vi "Facade.vi"(0 "Data In":T6, 2 "Display State In":T2={"Hierarchy"=[], "File/Directory Path"=path "", "Relative File Paths"=[], "Hide Undefined Channels"=FALSE, "Static File Structure"=FALSE, "Filtering"={"Filtered Groups"=[], "Group Filter Mode"=enum."Exclude", "Group Filter Regex?"=FALSE, "Filtered Channels"=[], "Channel Filter Mode"=enum."Exclude", "Channel Filter Regex?"=FALSE, "Filter Time Start"=timestamp(0 s since 1904-01-01), "Filter Time End"=timestamp(0 s since 1904-01-01), "Time Filter Mode"=enum."Include", "Time Filter Enabled"=FALSE}, "File Contents Tree"=refnum, "Properties Table"=refnum, "Loading Indicator"=refnum}, 3 "Container State":T5) -> (6 "Data Out":T6, 7 "Display State Out":T2={"Hierarchy"=[], "File/Directory Path"=path "", "Relative File Paths"=[], "Hide Undefined Channels"=FALSE, "Static File Structure"=FALSE, "Filtering"={"Filtered Groups"=[], "Group Filter Mode"=enum."Exclude", "Group Filter Regex?"=FALSE, "Filtered Channels"=[], "Channel Filter Mode"=enum."Exclude", "Channel Filter Regex?"=FALSE, "Filter Time Start"=timestamp(0 s since 1904-01-01), "Filter Time End"=timestamp(0 s since 1904-01-01), "Time Filter Mode"=enum."Include", "Time Filter Enabled"=FALSE}, "File Contents Tree"=refnum, "Properties Table"=refnum, "Loading Indicator"=refnum}, 8 "Action":T1)   [LabVIEW 2017, in "XTree.xctl"]
uses:
  <vilib>/addons/_NIFileIO/XTree/XTree.xctl
  <vilib>/addons/_NIFileIO/XTree/Data.ctl
  <vilib>/_xctls/Container State.ctl
  <vilib>/addons/_NIFileIO/XTree/State.ctl
  <vilib>/addons/_NIFileIO/XTree/Controls/Filter Settings.ctl
  <vilib>/addons/_NIFileIO/XTree/Controls/Filter Mode.ctl
  <vilib>/_xctls/Action.ctl
  <vilib>/Utility/miscctls.llb/LVRowAndColumnTypeDef.ctl
  <vilib>/_xctls/XControlSupport.lvlib
panel:
  out "Loading Indicator":string="Loading Tree Data..."
  in  "File Contents Tree":string(tree)
  out "Properties Table":string[][](table)
  # "1. Drop the controls that make up the appearance\nof the XControl here.\n\n2. Resize the window to fit the controls\n\n3. If the XControl is of fixed size,  make the \n window not resizable from VI Properties->Window Appearance.\n\n4. If you want the controls to automatically size when the XControl sizes, check  \"Scale all objects on front panel when window resizes\" in File->VI Properties->Window Size page.\n\n5. Show the block diagram and handle events for the controls on this panel."
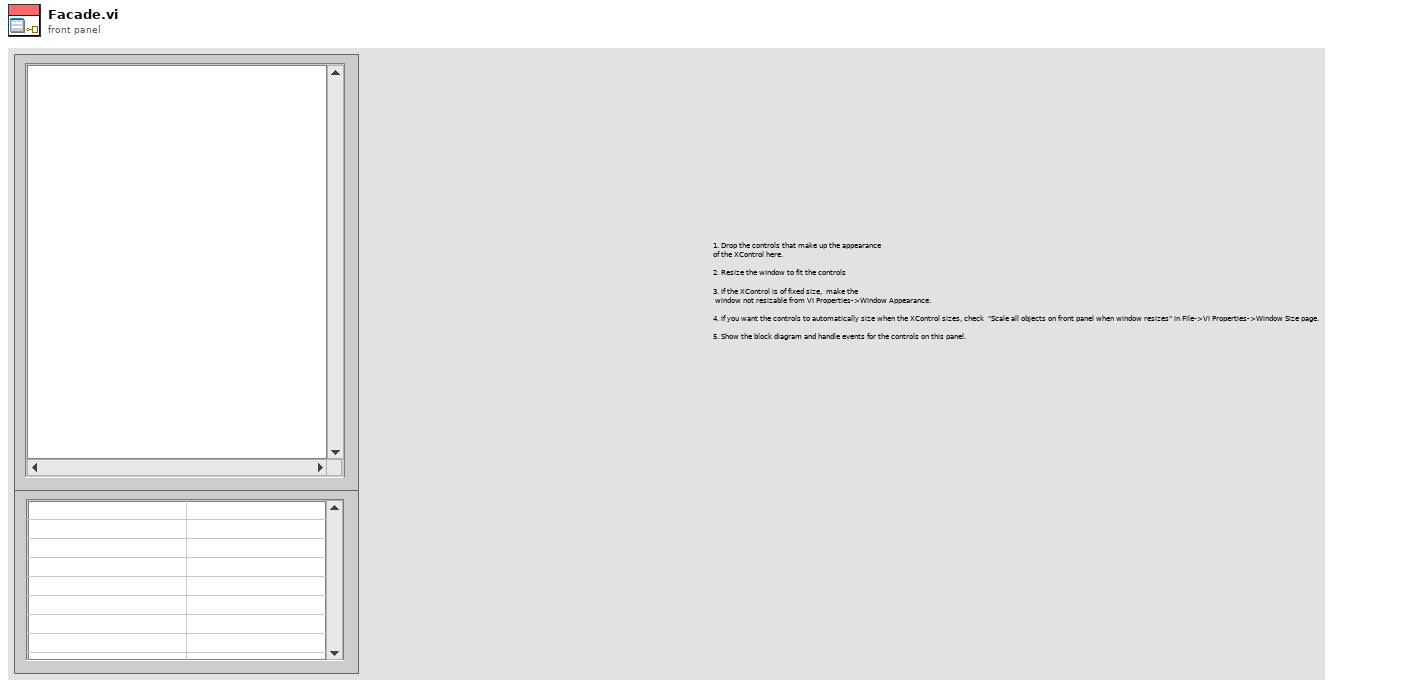
[diagram p1: front panel]
types:
  T1 = typedef "XControlSupport.lvlib/Action.ctl" = cluster{"Data Changed?":bool, "State Changed?":bool, "Action Name":string}
  T2 = typedef "XTree.xctl/State.ctl" = cluster{"Hierarchy":string[], "File/Directory Path":path, "Relative File Paths":string[], "Hide Undefined Channels":bool, "Static File Structure":bool, "Filtering":T3, "File Contents Tree":refnum<vi>, "Properties Table":refnum<vi>, "Loading Indicator":refnum<vi>}
  T3 = typedef "XTree.xctl/Filter Settings.ctl" = cluster{"Filtered Groups":string[], "Group Filter Mode":T4, "Group Filter Regex?":bool, "Filtered Channels":string[], "Channel Filter Mode":T4, "Channel Filter Regex?":bool, "Filter Time Start":timestamp, "Filter Time End":timestamp, "Time Filter Mode":T4, "Time Filter Enabled":bool}
  T4 = typedef "XTree.xctl/Filter Mode.ctl" = enum16{"Exclude", "Include"}
  T5 = typedef "XControlSupport.lvlib/Container State.ctl" = cluster{"Indicator?":bool, "Run Mode?":bool, " Refnum":refnum<vi>}
  T6 = typedef "XTree.xctl/Data.ctl" = variant
  T7 = typedef "LVRowAndColumnTypeDef.ctl" = cluster{"Row":i32, "Column":i32}
  T8 = enum16{"open", "open or create", "create or replace", "create", "open (read-only)"}
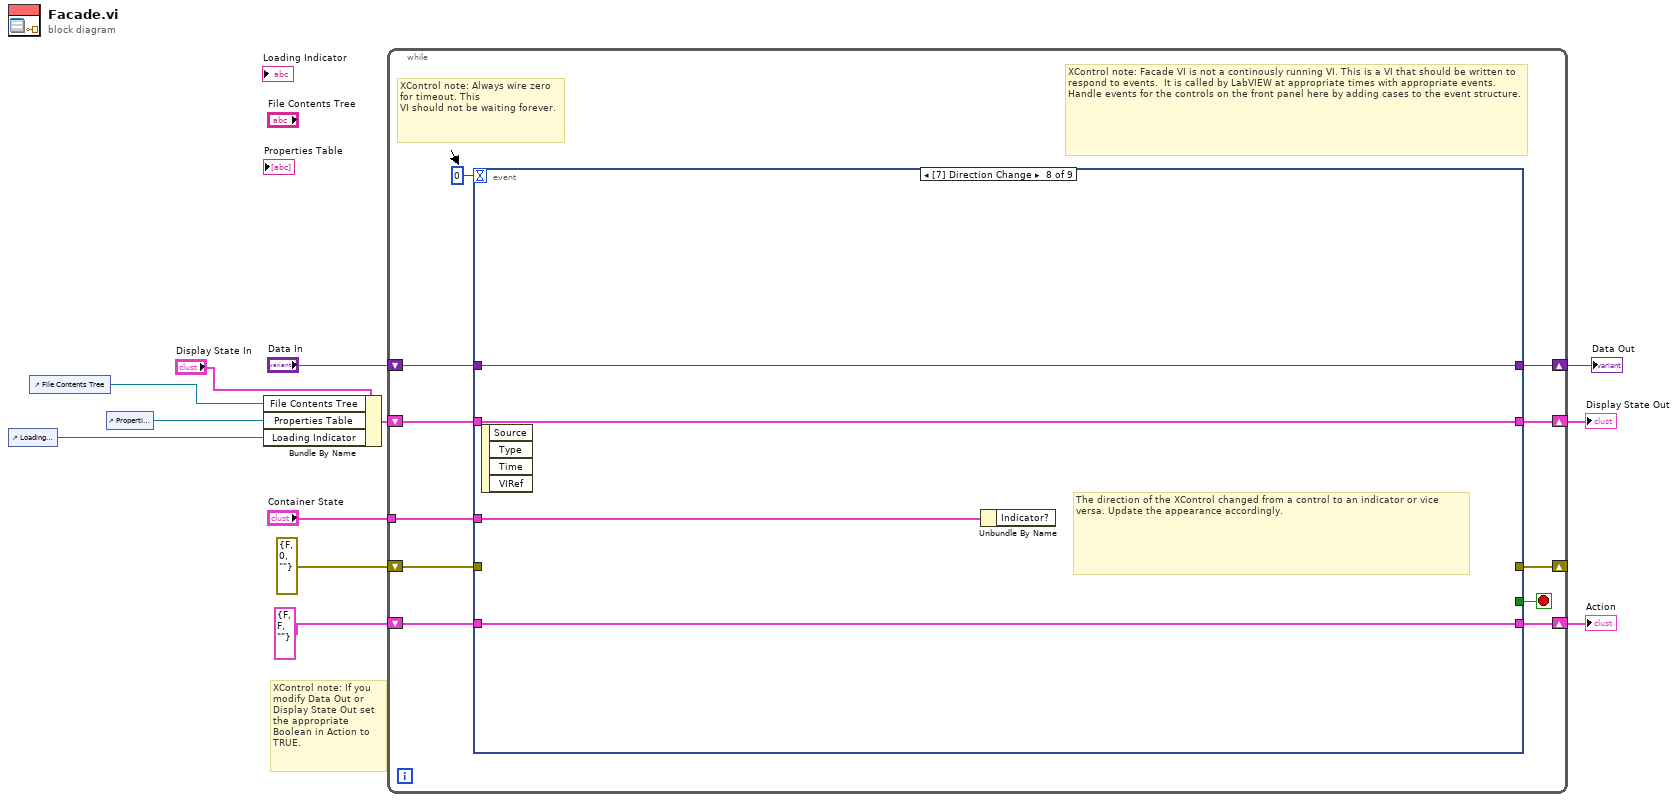
[diagram p0: block diagram]
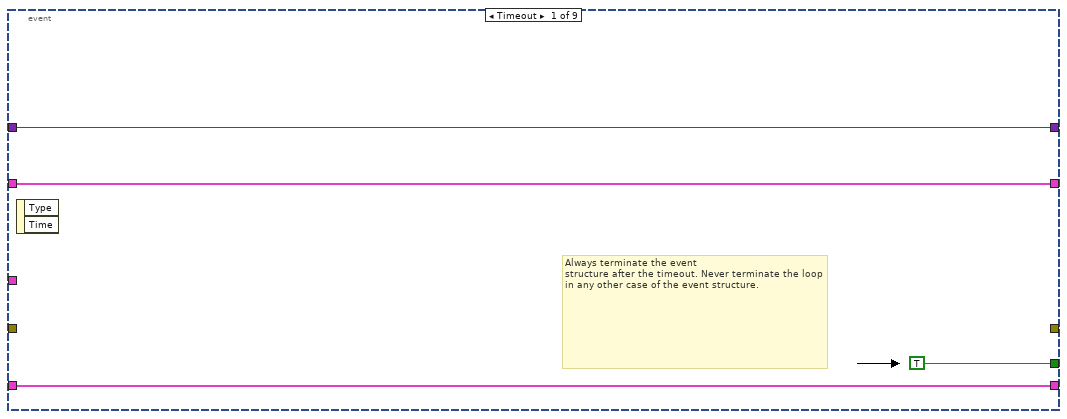
[diagram p2: hidden frame]
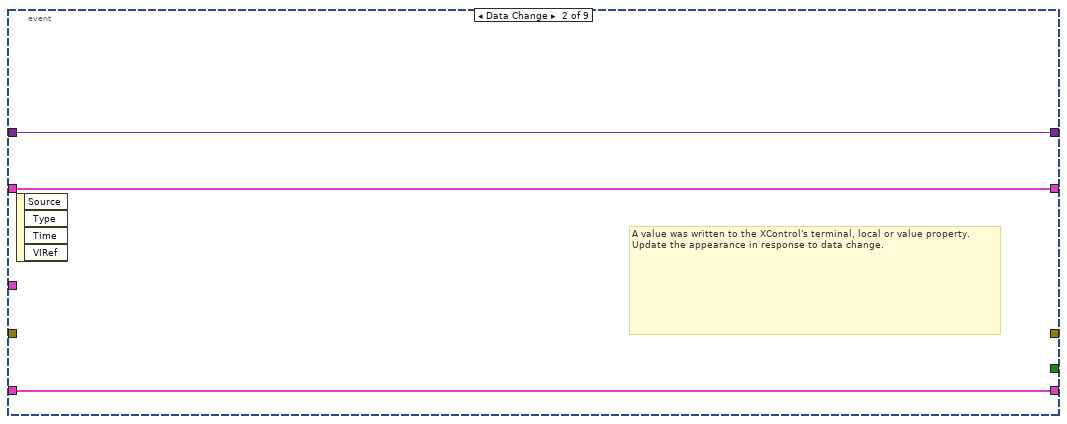
[diagram p3: hidden frame]
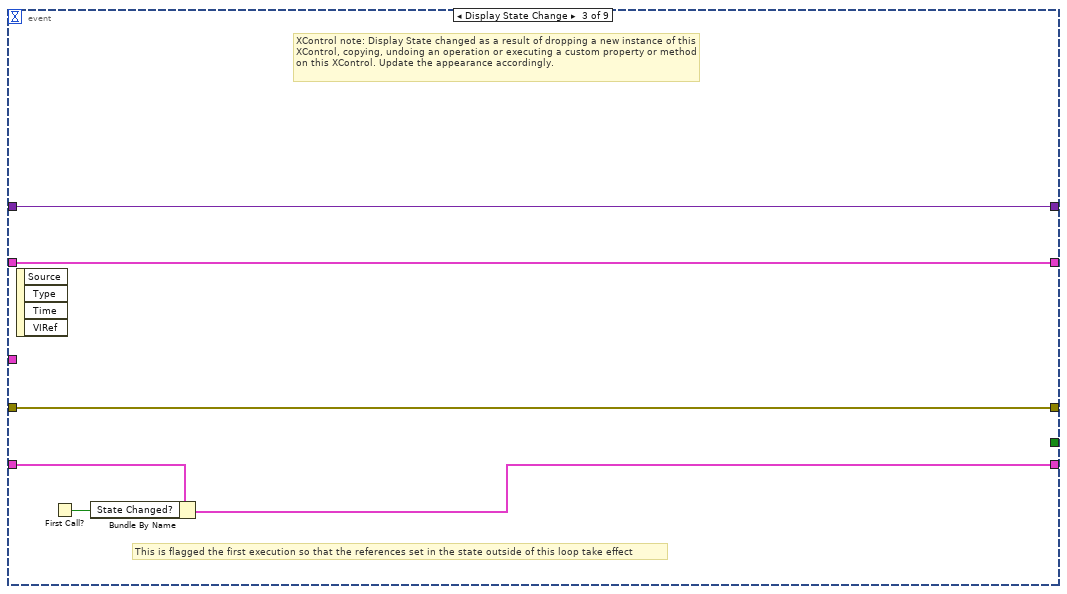
[diagram p4: hidden frame]
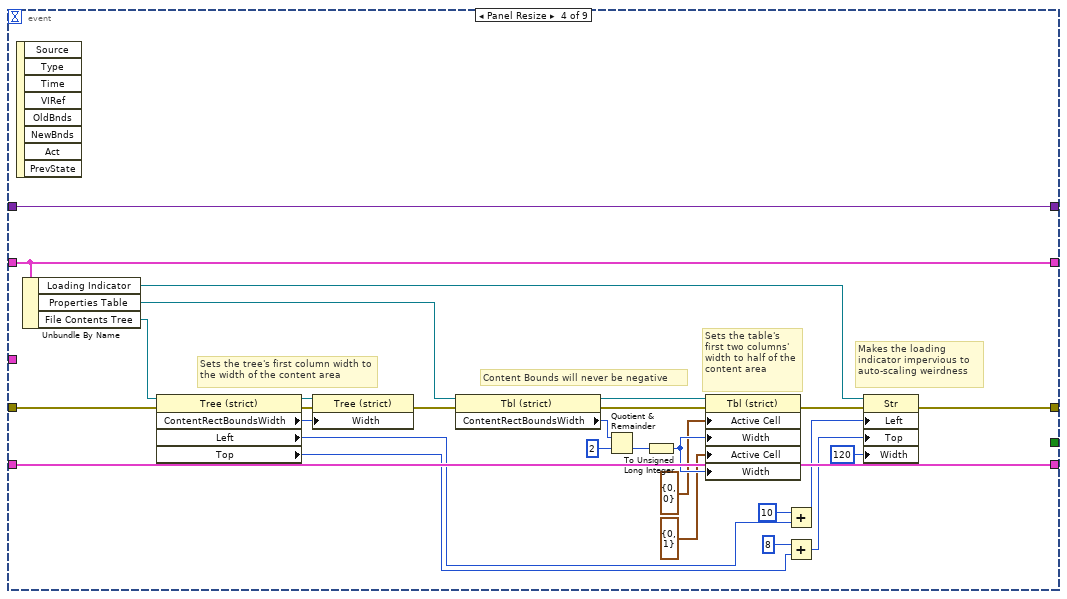
[diagram p5: hidden frame]
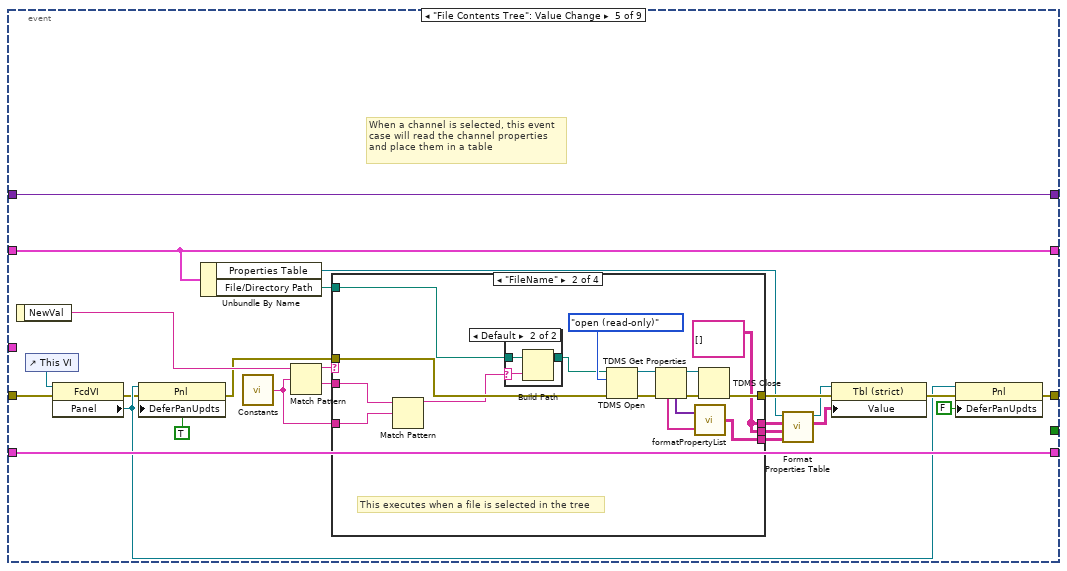
[diagram p6: hidden frame]
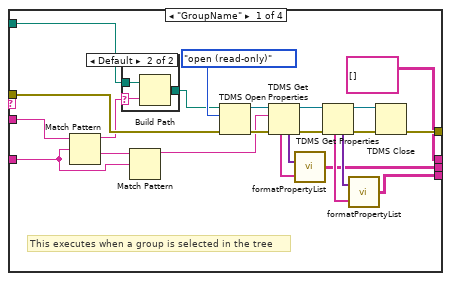
[diagram p7: hidden frame]
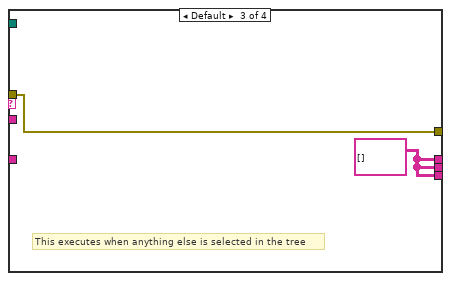
[diagram p10: hidden frame]
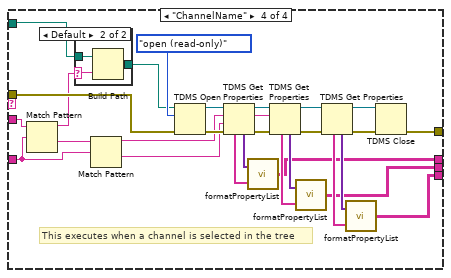
[diagram p11: hidden frame]
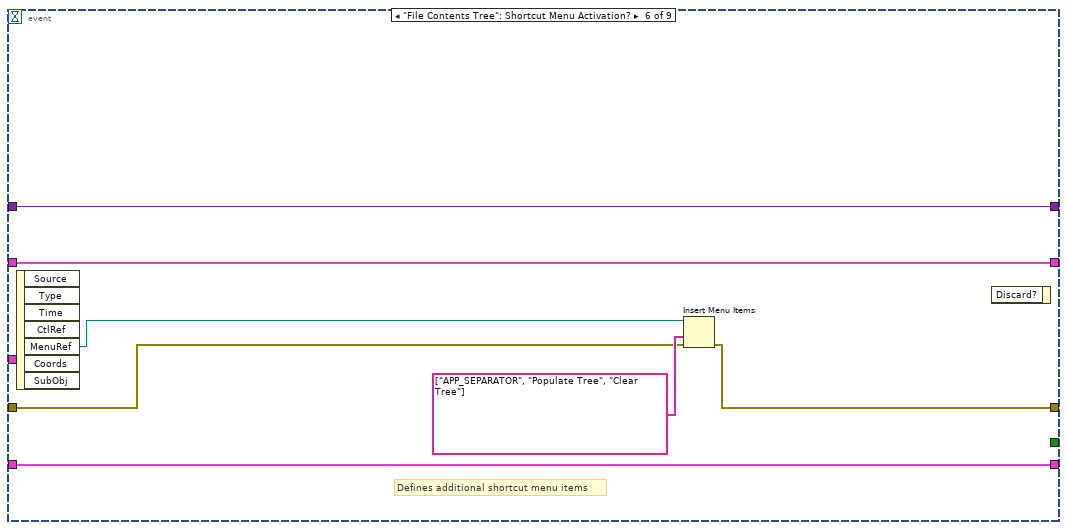
[diagram p13: hidden frame]
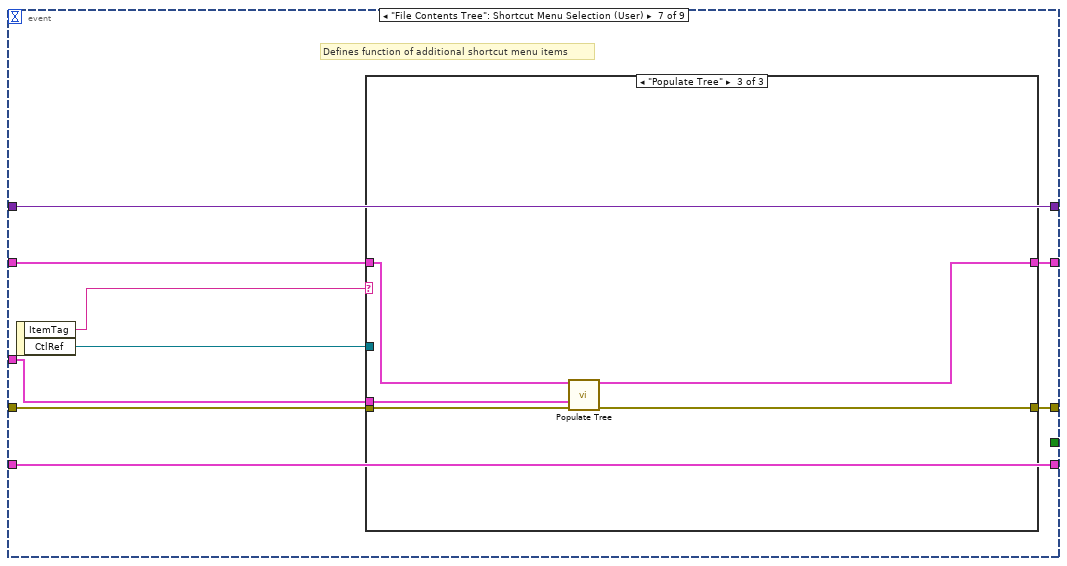
[diagram p14: hidden frame]
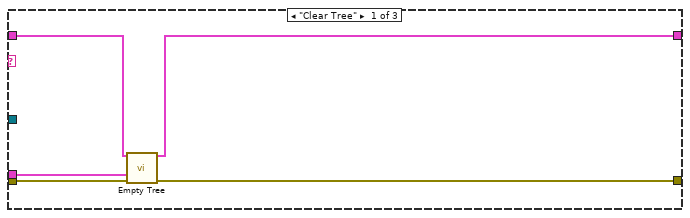
[diagram p15: hidden frame]
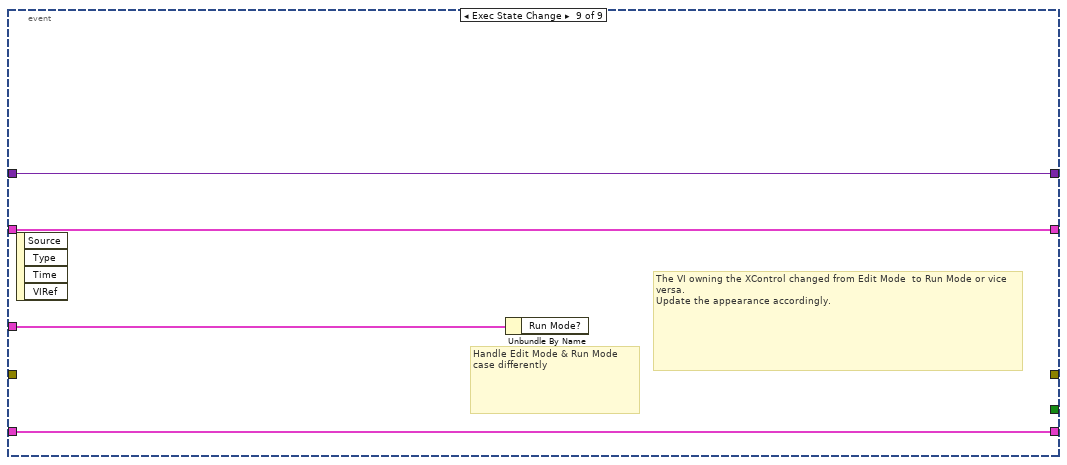
[diagram p17: hidden frame]
diagram:
  # "XControl note: If you modify Data Out or Display State Out set the appropriate Boolean in Action to TRUE."
  n1 = control-ref of="Loading Indicator"() -> (w1:refnum<vi>)
  n2 = control-ref of="File Contents Tree"() -> (w4:refnum<vi>)
  n3 = control-ref of="Properties Table"() -> (w5:refnum<vi>)
  n4 = Bundle By Name(cluster="Display State In", "File Contents Tree"=w4, "Properties Table"=w5, "Loading Indicator"=w1) -> (w2:T2)
  n5 = while {
    shift-right: [w22] -> w9
    shift-left: w2 -> [w23]
    tunnel: "Container State" -> [w19]
    shift-right: [w17] -> w12
    shift-left: "Data In" -> [w18]
    shift-right: [w15] -> w8
    shift-left: T1 {"Data Changed?"=FALSE, "State Changed?"=FALSE, "Action Name"=""} ("Action") -> [w16]
    shift-right: [w13] -> _
    shift-left: errorcluster {"status"=FALSE, "code"=0, "source"=""} ("error constant") -> [w14]
    stop <- w21 stop-if-true
    # "XControl note: Facade VI is not a continously running VI. This is a VI that should be written to respond to events.  It is called by LabVIEW at appropriate times with appropriate events. Handle events for the controls on the front panel here by adding cases to the event structure."
    # "XControl note: Always wire zero for timeout. This\nVI should not be waiting forever."
    n6 = event shown="[7] Direction Change" {
      selector: _ -> [_ _ _ _ _ _ _ _ _]
      dyn-events: _ -> [_ _ _ _ _ _ _ _ _]
      timeout: 0 -> [_ _ _ _ _ _ _ _ _]
      tunnel: w23 -> [w25 w29 w32 w52 w84 w177 w183 w201 w205]
      tunnel: [w25 w29 w32 w52 w84 w177 w180 w201 w205] -> w22
      tunnel: [TRUE _ _ _ _ _ _ _ _] -> w21
      tunnel: w19 -> [_ _ _ _ _ _ w182 w202 w206]
      tunnel: w18 -> [w24 w30 w35 w64 w88 w176 w186 w200 w204]
      tunnel: [w24 w30 w35 w64 w88 w176 w186 w200 w204] -> w17
      tunnel: [w26 w28 w33 w63 w75 w175 w185 w199 w203] -> w15
      tunnel: w16 -> [w26 w28 w36 w63 w75 w175 w185 w199 w203]
      tunnel: w14 -> [_ _ w34 w59 w66 w172 w184 _ _]
      tunnel: [_ _ w34 w45 w69 w171 w181 _ _] -> w13
      event Timeout {
        # "Always terminate the event\nstructure after the timeout. Never terminate the loop in any other case of the event structure."
        n7 = event-data() -> ()  [unwired: 1 in, 2 out]
      }
      event Data Change {
        # "A value was written to the XControl's terminal, local or value property.\nUpdate the appearance in response to data change."
        n8 = event-data() -> ()  [unwired: 1 in, 4 out]
      }
      event Display State Change {
        # "This is flagged the first execution so that the references set in the state outside of this loop take effect"
        # "XControl note: Display State changed as a result of dropping a new instance of this XControl, copying, undoing an operation or executing a custom property or method on this XControl. Update the appearance accordingly."
        n9 = event-data() -> ()  [unwired: 1 in, 4 out]
        n10 = First Call?() -> (First Call?: T/F=w31:bool)
        n11 = Bundle By Name(cluster=w36, "State Changed?"=w31) -> (w33:T1)
      }
      event Panel Resize {
        # "Makes the loading indicator impervious to auto-scaling weirdness"
        # "Sets the table's first two columns' width to half of the content area"
        # "Sets the tree's first column width to the width of the content area"
        # "Content Bounds will never be negative"
        n12 = event-data() -> ()  [unwired: 1 in, 8 out]
        n13 = Unbundle By Name(w52) -> ("Loading Indicator"=w37:refnum<vi>, "Properties Table"=w50:refnum<vi>, "File Contents Tree"=w51:refnum<vi>)
        n14 = property class="Tree (strict)"(reference=w51, error in=w59) -> (reference out=w61:refnum<vi>, error out=w62:errorcluster, "ContentRectBoundsWidth"=w60:i32, "Left"=w39:i32, "Top"=w42:i32)
        n15 = property class="Tree (strict)"(reference=w61, error in=w62, "Width"=w60) -> (error out=w58:errorcluster)  [unwired: 1 out]
        n16 = property class="Tbl (strict)"(reference=w50, error in=w58) -> (reference out=w55:refnum<vi>, error out=w54:errorcluster, "ContentRectBoundsWidth"=w57:i32)
        n17 = Quotient & Remainder(x=w57, y=2) -> (floor(x/y)=w53:i32)  [unwired: 1 out]
        n18 = To Unsigned Long Integer(number=w53) -> (unsigned 32bit integer=w49:u32)
        n19 = property class="Tbl (strict)"(reference=w55, error in=w54, "Active Cell"=T7 {"Row"=0, "Column"=0} ("Active Cell:Active Cell"), "Width"=w49, "Active Cell"=T7 {"Row"=0, "Column"=1} ("Active Cell:Active Cell"), "Width"=w49) -> (error out=w46:errorcluster)  [unwired: 1 out]
        n20 = Add(x=10 ("y"), y=w39) -> (x+y=w44:i32)
        n21 = Add(x=8, y=w42) -> (x+y=w43:i32)
        n22 = property class="Str"(reference=w37, error in=w46, "Left"=w44, "Top"=w43, "Width"=u32 120 ("Size:Width")) -> (error out=w45:errorcluster)  [unwired: 1 out]
      }
      event "File Contents Tree": Value Change {
        # "When a channel is selected, this event case will read the channel properties and place them in a table"
        n23 = event-data() -> ("NewVal"=w87:string)  [unwired: 1 in]
        n24 = control-ref of="This VI"() -> (w73:refnum<vi>)
        n25 = property class="FcdVI"(reference=w73, error in=w66) -> (error out=w65:errorcluster, "Panel"=w67:refnum<vi>)  [unwired: 1 out]
        n26 = property class="Pnl"(reference=w67, error in=w65, "DeferPanUpdts"=TRUE ("Defer Panel Updates")) -> (error out=w72:errorcluster)  [unwired: 1 out]
        n27 = Unbundle By Name(w84) -> ("Properties Table"=w81:refnum<vi>, "File/Directory Path"=w74:path)
        n28 = call <vilib>:"Constants.vi"() -> ("String Delimeter"=w85:string)  [unwired: 5 in]
        n29 = Match Pattern(string=w87, regular expression=w85) -> (before substring=w83:string, after substring=w86:string)  [unwired: 1 in, 2 out]
        n30 = case shown="\"FileName\"" w83 {
          tunnel: w86 -> [w108 w128 _ w161]
          tunnel: w85 -> [w101 w127 _ w152]
          tunnel: w74 -> [w91 w118 _ w140]
          tunnel: w72 -> [w92 w119 w137 w141]
          tunnel: [w107 w122 w137 w162] -> w82
          tunnel: [string[][] [] ("strings") w120 w136 w144] -> w79
          tunnel: [w95 w120 w136 w143] -> w78
          tunnel: [w94 w121 w136 w142] -> w77
          frame "GroupName" {
            # "This executes when a group is selected in the tree"
            n31 = Match Pattern(string=w108, regular expression=w101) -> (before substring=w90:string, after substring=w102:string)  [unwired: 1 in, 2 out]
            n32 = case shown="Default" w90 {
              selector: w90 -> [_ w113]
              tunnel: w91 -> [w112 w115]
              tunnel: [w112 w114] -> w89
              frame "" {
              }
              frame Default {
                n33 = Build Path(base path=w115, name or relative path=w113) -> (appended path=w114:path)
              }
            }
            n34 = Match Pattern(string=w102, regular expression=w101) -> (before substring=w100:string)  [unwired: 1 in, 3 out]
            n35 = TDMS Open(8:w92, 10:T8."open (read-only)" ("operation (0:open)"), 11:w89) -> (0:w110:errorcluster, 3:w109:refnum<k34>)  [unwired: 4 in]
            n36 = TDMS Get Properties(8:w110, 10:w100, 11:w109) -> (0:w104:errorcluster, 3:w106:refnum<k34>, 4:w98:variant[], 6:w99:string[])  [unwired: 3 in, 2 out]
            n37 = call <vilib>:"formatPropertyList.vi"("property names"=w99, "property values"=w98) -> ("strings"=w95:string[][])
            n38 = TDMS Get Properties(8:w104, 11:w106) -> (0:w103:errorcluster, 3:w105:refnum<k34>, 4:w96:variant[], 6:w97:string[])  [unwired: 4 in, 2 out]
            n39 = call <vilib>:"formatPropertyList.vi"("property names"=w97, "property values"=w96) -> ("strings"=w94:string[][])
            n40 = TDMS Close(8:w103, 11:w105) -> (0:w107:errorcluster)  [unwired: 1 out]
          }
          frame "FileName" {
            w120 = string[][] [] ("strings")
            # "This executes when a file is selected in the tree"
            n41 = Match Pattern(string=w128, regular expression=w127) -> (before substring=w117:string)  [unwired: 1 in, 3 out]
            n42 = case shown="Default" w117 {
              selector: w117 -> [_ w133]
              tunnel: w118 -> [w132 w135]
              tunnel: [w132 w134] -> w116
              frame "" {
              }
              frame Default {
                n43 = Build Path(base path=w135, name or relative path=w133) -> (appended path=w134:path)
              }
            }
            n44 = TDMS Open(8:w119, 10:T8."open (read-only)" ("operation (0:open)"), 11:w116) -> (0:w130:errorcluster, 3:w129:refnum<k34>)  [unwired: 4 in]
            n45 = TDMS Get Properties(8:w130, 11:w129) -> (0:w126:errorcluster, 3:w125:refnum<k34>, 4:w124:variant[], 6:w123:string[])  [unwired: 4 in, 2 out]
            n46 = call <vilib>:"formatPropertyList.vi"("property names"=w123, "property values"=w124) -> ("strings"=w121:string[][])
            n47 = TDMS Close(8:w126, 11:w125) -> (0:w122:errorcluster)  [unwired: 1 out]
          }
          frame Default {
            w136 = string[][] [] ("strings")
            # "This executes when anything else is selected in the tree"
          }
          frame "ChannelName" {
            # "This executes when a channel is selected in the tree"
            n48 = Match Pattern(string=w161, regular expression=w152) -> (before substring=w139:string, after substring=w160:string)  [unwired: 1 in, 2 out]
            n49 = case shown="Default" w139 {
              selector: w139 -> [_ w168]
              tunnel: w140 -> [w167 w170]
              tunnel: [w167 w169] -> w138
              frame "" {
              }
              frame Default {
                n50 = Build Path(base path=w170, name or relative path=w168) -> (appended path=w169:path)
              }
            }
            n51 = Match Pattern(string=w160, regular expression=w152) -> (before substring=w163:string, after substring=w151:string)  [unwired: 1 in, 2 out]
            n52 = TDMS Open(8:w141, 10:T8."open (read-only)" ("operation (0:open)"), 11:w138) -> (0:w165:errorcluster, 3:w164:refnum<k34>)  [unwired: 4 in]
            n53 = TDMS Get Properties(8:w165, 9:w151, 10:w163, 11:w164) -> (0:w156:errorcluster, 2:w153:string, 3:w159:refnum<k34>, 4:w150:variant[], 6:w149:string[])  [unwired: 2 in, 1 out]
            n54 = call <vilib>:"formatPropertyList.vi"("property names"=w149, "property values"=w150) -> ("strings"=w144:string[][])
            n55 = TDMS Get Properties(8:w156, 10:w153, 11:w159) -> (0:w155:errorcluster, 3:w158:refnum<k34>, 4:w147:variant[], 6:w148:string[])  [unwired: 3 in, 2 out]
            n56 = call <vilib>:"formatPropertyList.vi"("property names"=w148, "property values"=w147) -> ("strings"=w143:string[][])
            n57 = TDMS Get Properties(8:w155, 11:w158) -> (0:w154:errorcluster, 3:w157:refnum<k34>, 4:w145:variant[], 6:w146:string[])  [unwired: 4 in, 2 out]
            n58 = call <vilib>:"formatPropertyList.vi"("property names"=w146, "property values"=w145) -> ("strings"=w142:string[][])
            n59 = TDMS Close(8:w154, 11:w157) -> (0:w162:errorcluster)  [unwired: 1 out]
          }
        }
        n60 = call <vilib>:"Format Properties Table.vi"("File Properties"=w77, "Group Properties"=w78, "Channel Properties"=w79, "Properties Table In"=w81) -> ("Properties Out"=w76:string[][], "Properties Table Out"=w80:refnum<vi>)  [unwired: 6 in]
        n61 = property class="Tbl (strict)"(reference=w80, error in=w82, "Value"=w76) -> (error out=w70:errorcluster)  [unwired: 1 out]
        n62 = property class="Pnl"(reference=w67, error in=w70, "DeferPanUpdts"=FALSE ("Defer Panel Updates")) -> (error out=w69:errorcluster)  [unwired: 1 out]
      }
      event "File Contents Tree": Shortcut Menu Activation? {
        # "Defines additional shortcut menu items"
        n63 = event-data() -> ("MenuRef"=w173:refnum<k9>)  [unwired: 1 in, 6 out]
        n64 = Insert Menu Items(6:w172, 7:string[] ["APP_SEPARATOR", "Populate Tree", "Clear Tree"], 9:w173) -> (0:w171:errorcluster)  [unwired: 3 in, 2 out]
        n65 = event-data() -> ()  [unwired: 2 in, 1 out]
      }
      event "File Contents Tree": Shortcut Menu Selection (User) {
        # "Defines function of additional shortcut menu items"
        n66 = event-data() -> ("ItemTag"=w178:string, "CtlRef"=w179:refnum<vi>)  [unwired: 1 in]
        n67 = case shown="\"Populate Tree\"" w178 {
          tunnel: w184 -> [w191 w192 w196]
          tunnel: w183 -> [w187 w193 w198]
          tunnel: w182 -> [w189 _ w197]
          tunnel: [w190 w192 w195] -> w181
          tunnel: [w188 w193 w194] -> w180
          tunnel: w179 -> [_ _ _]
          frame "Clear Tree" {
            n68 = call <vilib>:"Empty Tree.vi"("Display State In"=w187, "Container State"=w189, "error in (no error)"=w191) -> ("Display State Out"=w188:T2, "error out"=w190:errorcluster)  [unwired: 11 in]
          }
          frame Default {
          }
          frame "Populate Tree" {
            n69 = call <vilib>:"Populate Tree.vi"("Display State In"=w198, "Container State"=w197, "error in (no error)"=w196) -> ("Display State Out"=w194:T2, "error out"=w195:errorcluster)  [unwired: 11 in]
          }
        }
      }
      event Direction Change {
        # "The direction of the XControl changed from a control to an indicator or vice versa. Update the appearance accordingly."
        n70 = event-data() -> ()  [unwired: 1 in, 4 out]
        n71 = Unbundle By Name(w202) -> ()  [unwired: 1 out]
      }
      event Exec State Change {
        # "The VI owning the XControl changed from Edit Mode  to Run Mode or vice versa.\nUpdate the appearance accordingly."
        # "Handle Edit Mode & Run Mode\ncase differently"
        n72 = event-data() -> ()  [unwired: 1 in, 4 out]
        n73 = Unbundle By Name(w206) -> ()  [unwired: 1 out]
      }
    }
  }
  "Display State Out" <- w9
  "Data Out" <- w12
  "Action" <- w8
